vi "start function.vi"(8 "running command array":string[][](array[string]), 9 "command in":string[](array[string]), 10 "old sensor datas":T1, 11 "sensor datas":T1) -> (3 "start?":bool)   [LabVIEW 2011]
panel:
  in  "error in (no error)":errorcluster
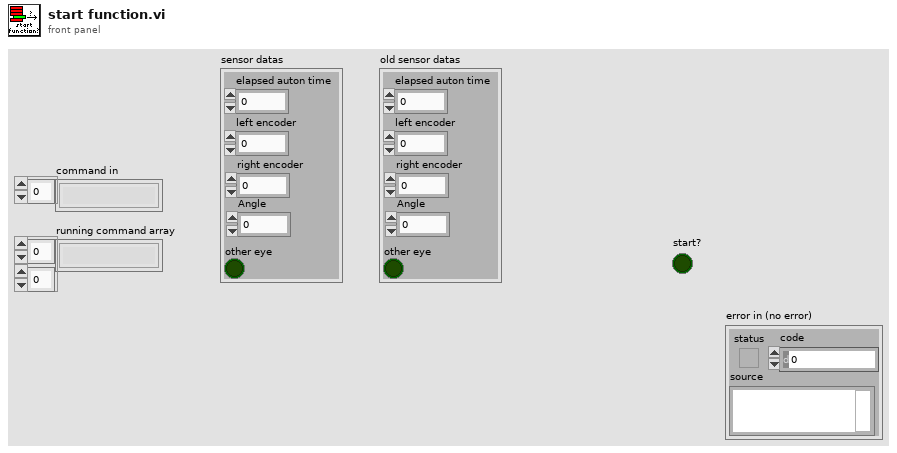
[diagram p1: front panel]
types:
  T1 = cluster{"elapsed auton time":dbl, "left encoder":dbl, "other eye":bool, "right encoder":dbl, "Angle":dbl}
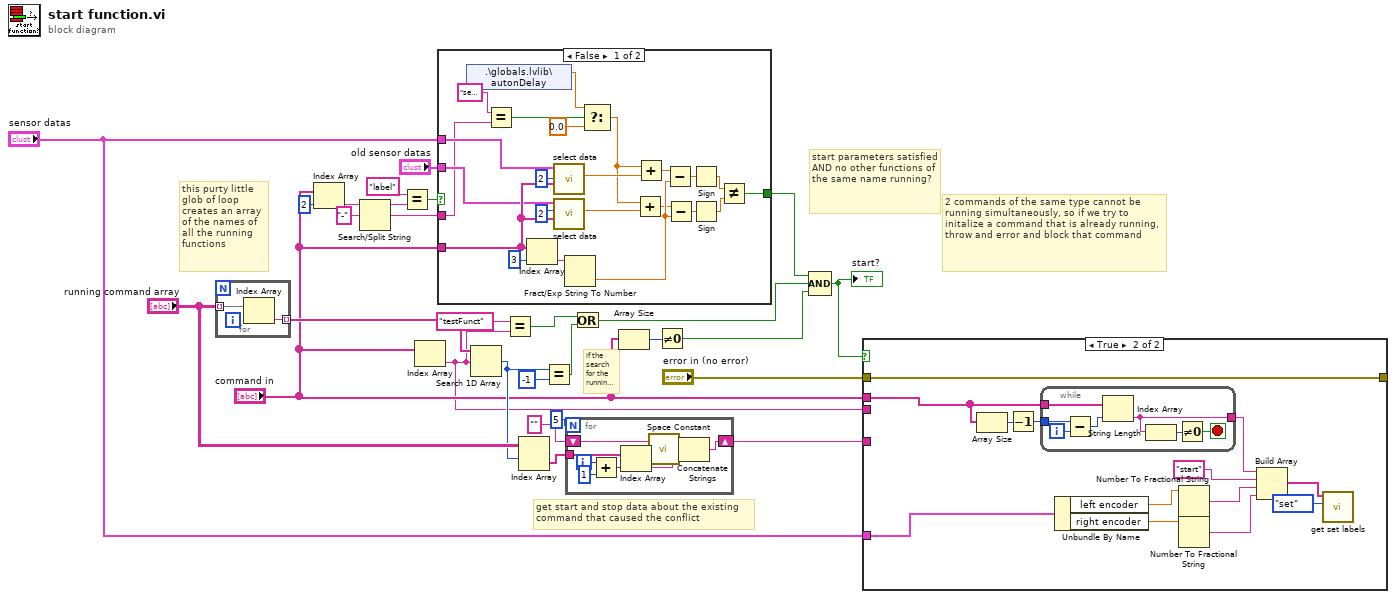
[diagram p0: block diagram]
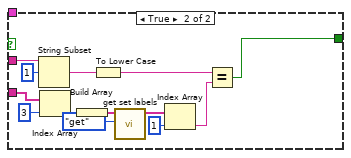
[diagram p2: hidden frame]
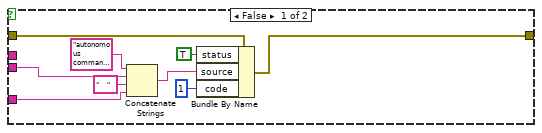
[diagram p3: hidden frame]
diagram:
  # "get start and stop data about the existing command that caused the conflict"
  # "if the search for the running function returns a -1, it was not found in the array of running functions and we can start this one."
  # "start parameters satisfied AND no other functions of the same name running?"
  # "this purty little glob of loop creates an array of the names of all the running functions"
  # "2 commands of the same type cannot be running simultaneously, so if we try to initalize a command that is already running,  throw and error and block that command"
  n1 = for {
    tunnel: "running command array" -> [w30] mode=indexing
    tunnel: [w29] -> w28 mode=indexing
    n2 = Index Array(array=w30) -> (element=w29:string)  [unwired: 1 in]
  }
  n3 = Index Array(array="command in", index=2) -> (element=w19:string)
  n4 = Search/Split String(string=w19, search string/char (-)="-") -> (substring before match=w16:string, match + rest of string=w13:string)  [unwired: 1 in, 1 out]
  n5 = Equal?(x="label", y=w16) -> (x = y?=w14:bool)
  n6 = Index Array(array="command in") -> (element=w5:string)  [unwired: 1 in]
  n7 = case shown="False" w14 {
    tunnel: [w45 w56] -> w12
    tunnel: "command in" -> [w43 w64]
    tunnel: w13 -> [w36 w66]
    tunnel: "sensor datas" -> [w42 _]
    tunnel: "old sensor datas" -> [w41 _]
    frame False {
      n8 = shared-variable ".\\globals.lvlib\\autonDelay"() -> (w33:dbl)  [unwired: 1 in, 1 out]
      n9 = Equal?(x="setShooterRPMNoDelay", y=w36) -> (x = y?=w34:bool)
      n10 = Index Array(array=w43, index=3) -> (element=w52:string)
      n11 = call "select data.vi"("command and parameters in"=w43, "index"=u8 2, "sensor datas"=w42) -> ("accessed value"=w39:dbl)  [unwired: 8 in]
      n12 = call "select data.vi"("command and parameters in"=w43, "index"=u8 2, "sensor datas"=w41) -> ("accessed value"=w37:dbl)  [unwired: 8 in]
      n13 = Fract/Exp String To Number(string=w52) -> (number=w50:dbl)  [unwired: 3 in, 1 out]
      n14 = Select(t=w33, s=w34, f=0.0) -> (s? t:f=w31:dbl)
      n15 = Add(x=w31, y=w37) -> (x+y=w38:dbl)
      n16 = Add(x=w31, y=w39) -> (x+y=w40:dbl)
      n17 = Subtract(x=w40, y=w50) -> (x-y=w49:dbl)
      n18 = Subtract(x=w38, y=w50) -> (x-y=w48:dbl)
      n19 = Sign(1:w49) -> (0:w47:dbl)
      n20 = Sign(1:w48) -> (0:w46:dbl)
      n21 = Not Equal?(x=w47, y=w46) -> (x != y?=w45:bool)
    }
    frame True {
      n22 = String Subset(string=w66, offset (0)=1) -> (substring=w60:string)  [unwired: 1 in]
      n23 = Index Array(array=w64, index=3) -> (element=w62:string)
      n24 = Build Array(w62) -> (w61:string[])
      n25 = To Lower Case(string=w60) -> (all lower case string=w59:string)
      n26 = call "get set labels.vi"("option in"=enum16{"get", "set", "remove", "set end"}."get", "label in"=w61) -> ("label out"=w58:string[])  [unwired: 9 in]
      n27 = Index Array(array=w58, index=1) -> (element=w57:string)
      n28 = Equal?(x=w59, y=w57) -> (x = y?=w56:bool)
    }
  }
  n29 = Search 1D Array(1D array=w28, element=w5) -> (index of element=w25:i32)  [unwired: 1 in]
  n30 = Equal?(x="testFunct", y=w5) -> (x = y?=w3:bool)
  n31 = Index Array(array="running command array", index (row)=w25) -> (element=w23:string[])  [unwired: 1 in]
  n32 = Equal?(x=w25, y=-1) -> (x = y?=w7:bool)
  n33 = for {
    N: 5 -> [_]
    tunnel: w23 -> [w74]
    shift-right: [w70] -> w21
    shift-left: "" -> [w69]
    i -> [w73]
    n34 = Add(x=w73, y=1) -> (x+y=w72:i32)
    n35 = Index Array(array=w74, index=w72) -> (element=w67:string)
    n36 = call <vilib>:"Space Constant.vi"() -> ("String"=w68:string)
    n37 = Concatenate Strings(w69, w68, w67) -> (w70:string)
  }
  n38 = Or(x=w3, y=w7) -> (x .or. y?=w6:bool)
  n39 = Array Size(array="command in") -> (size(s)=w9:i32)
  n40 = Not Equal To 0?(x=w9) -> (x != 0?=w8:bool)
  n41 = Compound Arithmetic op=AND(w12, w6, w8) -> (w11:bool)
  "start?" <- w11
  n42 = case shown="True" w11 {
    tunnel: "error in (no error)" -> [w83 w96]
    tunnel: [w81 w96] -> _
    tunnel: w21 -> [w76 _]
    tunnel: w5 -> [w78 _]
    tunnel: "command in" -> [_ w86]
    tunnel: "sensor datas" -> [_ w85]
    frame False {
      n43 = Concatenate Strings("autonomous command onflict caused by new " ("string"), w78, "    " ("string"), w76) -> (w75:string)
      n44 = Bundle By Name(cluster=w83, "status"=TRUE, "source"=w75, "code"=1) -> (w81:errorcluster)
    }
    frame True {
      n45 = Array Size(array=w86) -> (size(s)=w89:i32)
      n46 = Decrement(x=w89) -> (x-1=w88:i32)
      n47 = while {
        tunnel: w86 -> [w101]
        tunnel: w88 -> [w102]
        tunnel: [w98] -> w87
        i -> [w103]
        stop <- w97 stop-if-true
        n48 = Subtract(x=w102, y=w103) -> (x-y=w100:i32)
        n49 = Index Array(array=w101, index=w100) -> (element=w98:string)
        n50 = String Length(string=w98) -> (length=w99:i32)
        n51 = Not Equal To 0?(x=w99) -> (x != 0?=w97:bool)
      }
      n52 = Unbundle By Name(w85) -> ("left encoder"=w95:dbl, "right encoder"=w94:dbl)
      n53 = Number To Fractional String(number=w95) -> (F-format string=w93:string)  [unwired: 3 in]
      n54 = Number To Fractional String(number=w94) -> (F-format string=w92:string)  [unwired: 3 in]
      n55 = Build Array(w87, "start" ("element"), w93, w92) -> (w90:string[])
      n56 = call "get set labels.vi"("option in"=enum16{"get", "set", "remove", "set end"}."set", "label in"=w90) -> ()  [unwired: 9 in, 1 out]
    }
  }
